vi "Create New PropertyObject.vi"(11 "Sequence Context":refnum<k7>) -> (0 "error out":errorcluster)   [LabVIEW 2011]
doc: "This VI creates a new PropertyObject using the NewPropertyObject() method and is then inserted as a Local variable with the name \"MyString\"."
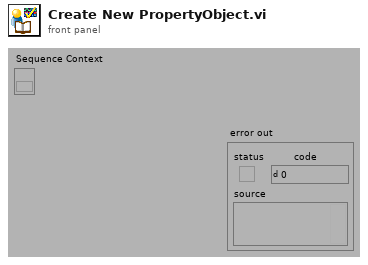
[diagram p1: front panel]
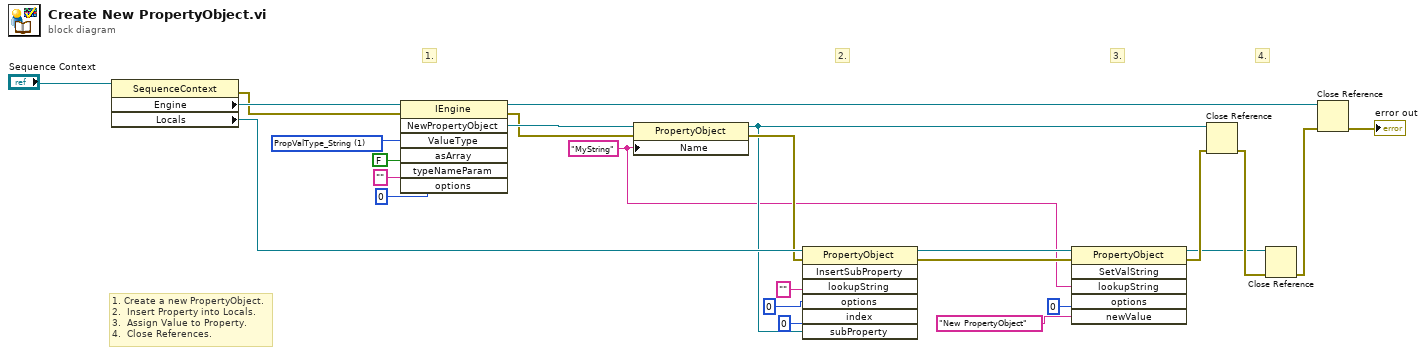
[diagram p0: block diagram]
diagram:
  w5 = "MyString" ("Name")
  w23 = 1 items=["PropValType_Container", "PropValType_String", "PropValType_Boolean", "PropValType_Number", "PropValType_NamedType", "PropValType_Reference", "PropValType_Array"] ("ValueType")
  # "4."
  # "3."
  # "2."
  # "1. Create a new PropertyObject.\n2.  Insert Property into Locals.\n3.  Assign Value to Property.\n4.  Close References."
  # "1."
  n1 = property class="SequenceContext"(reference="Sequence Context") -> (error out=w24:errorcluster, "Engine"=w25:refnum<k7>, "Locals"=w17:refnum<k7>)  [unwired: 1 in, 1 out]
  n2 = invoke class="IEngine" method="NewPropertyObject"(reference=w25, error in=w24, "ValueType"=w23, "asArray"=FALSE, "typeNameParam"="", "options"=0) -> (reference out=w10:refnum<k7>, error out=w18:errorcluster, "NewPropertyObject"=w19:refnum<k7>)  [unwired: 1 in, 4 out]
  n3 = property class="PropertyObject"(reference=w19, error in=w18, "Name"=w5) -> (reference out=w12:refnum<k7>, error out=w16:errorcluster)
  n4 = invoke class="PropertyObject" method="InsertSubProperty"(reference=w17, error in=w16, "lookupString"="", "options"=0, "index"=0, "subProperty"=w12) -> (reference out=w7:refnum<k7>, error out=w6:errorcluster)  [unwired: 1 in, 5 out]
  n5 = invoke class="PropertyObject" method="SetValString"(reference=w7, error in=w6, "lookupString"=w5, "options"=0, "newValue"="New PropertyObject") -> (reference out=w1:refnum<k7>, error out=w2:errorcluster)  [unwired: 1 in, 4 out]
  n6 = Close Reference(reference=w12, error in (no error)=w2) -> (error out=w11:errorcluster)
  n7 = Close Reference(reference=w1, error in (no error)=w11) -> (error out=w9:errorcluster)
  n8 = Close Reference(reference=w10, error in (no error)=w9) -> (error out=→"error out":errorcluster)
